vi "Tosca-2P Synchronization Simulator.vi"() -> ()   [LabVIEW 2020]
uses:
  <resource>/objmgr/daqmx.rc
  <vilib>/DAQmx/write.llb/DAQmx Write (Analog 2D DBL NChan NSamp).vi
  <vilib>/DAQmx/configure/timing.llb/DAQmx Timing (Sample Clock).vi
  <vilib>/DAQmx/create/channels.llb/DAQmx Create Channel (AO-Voltage-Basic).vi
  Signal Synthesis VIs/Waveform VIs/Pulse Train VIs/Pulse Polarity.ctl
  Signal Synthesis VIs/3rd Generation/Waveform VIs/Pulse Train VIs/Pulse Train.Properties.ctl
panel:
  in  "Nominal \"stim\" rate":dbl=1.0 format="%0.2f"
  in  "device":tag="PXI1Slot5"
  in  "Drift rate (us/s)":dbl format="%0.2f"
  in  "stop":bool
  in  "Buffer (s)":dbl=0.2 format="%0.2f"
  in  "Fs (Hz)":dbl=100000.0 format="%0.2f"
  in  "Pulse Train.Properties":T1={"Pulse width (us)"=10000.0, "Pulse rate (Hz)"=29.98, "Gap (ms)"=0.0, "Polarity"=enum."POS", "Asynch"=FALSE}
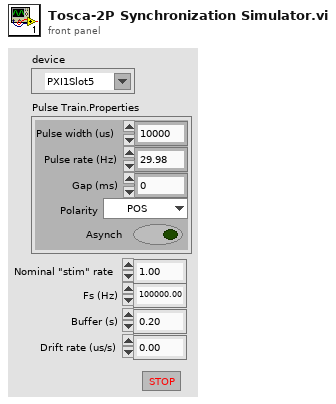
[diagram p1: front panel]
types:
  T1 = typedef "Pulse Train.Properties.ctl" = cluster{"Pulse width (us)":dbl, "Pulse rate (Hz)":dbl, "Gap (ms)":dbl, "Polarity":T2, "Asynch":bool}
  T2 = typedef "Pulse Polarity.ctl" = enum16{"POS", "NEG", "POS-NEG", "NEG-POS"}
  T3 = typedef "Pulse Train-Continuous State.ctl" = cluster{"Template":dbl[], "Nperiod":i32, "Index":i32, "Pulse Rate (Hz)":dbl, "Phase (cycles)":dbl, "Noff":i32}
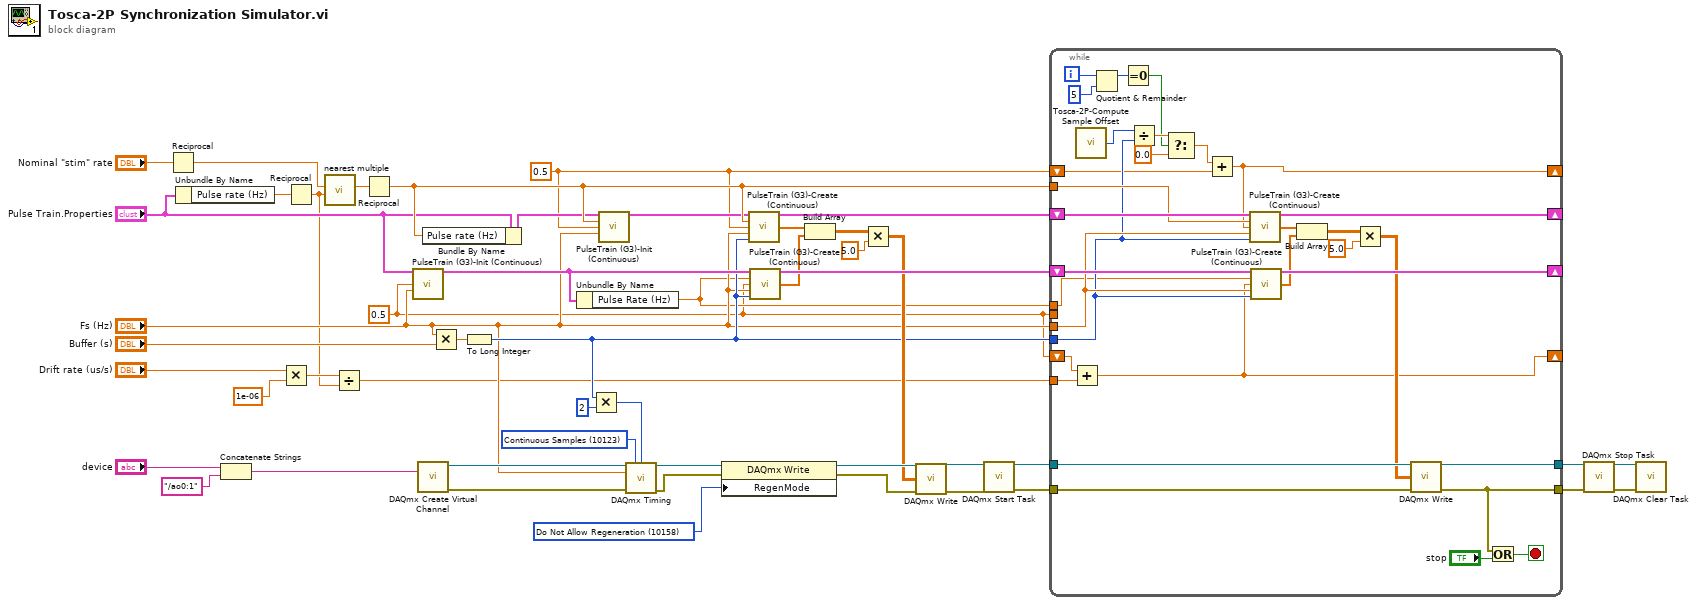
[diagram p0: block diagram]
diagram:
  w4 = 0.5 ("Start Phase (cycles)")
  w7 = 0.5 ("Start Phase (cycles)")
  w43 = 10158 items=["Allow Regeneration"=10097, "Do Not Allow Regeneration"=10158] ("RegenMode")
  w47 = 10123 items=["Finite Samples"=10178, "Continuous Samples"=10123, "Hardware Timed Single Point"=12522] ("sample mode")
  n1 = Reciprocal(x="Nominal \"stim\" rate") -> (1/x=w14:dbl)
  n2 = Unbundle By Name("Pulse Train.Properties") -> ("Pulse rate (Hz)"=w15:dbl)
  n3 = Concatenate Strings("device", "/ao0:1") -> (w23:string)
  n4 = Multiply(x="Drift rate (us/s)", y=1e-06) -> (x*y=w3:dbl)
  n5 = Reciprocal(x=w15) -> (1/x=w2:dbl)
  n6 = call "nearest multiple.vi"("y"=w2, "x"=w14) -> ("round(x/y)*y"=w13:dbl)  [unwired: 7 in, 2 out]
  n7 = Divide(x=w3, y=w2) -> (x/y=w1:dbl)
  n8 = Reciprocal(x=w13) -> (1/x=w12:dbl)
  n9 = call "PulseTrain (G3)-Init (Continuous).vi"("Pulse Train Params"="Pulse Train.Properties", "Start Phase (cycles)"=w4, "Fs (Hz)"="Fs (Hz)") -> ("Initial State"=w40:T3)  [unwired: 11 in, 1 out]
  n10 = call-poly <vilib>:"DAQmx Create Virtual Channel.vi"("physical channels"=w23) -> ("task out"=w49:refnum<k21>, "error out"=w48:errorcluster)  [unwired: 13 in]
  n11 = Bundle By Name(cluster="Pulse Train.Properties", "Pulse rate (Hz)"=w12) -> (w9:T1)
  n12 = Multiply(x="Fs (Hz)", y="Buffer (s)") -> (x*y=w46:dbl)
  n13 = To Long Integer(number=w46) -> (32bit integer=w17:i32)
  n14 = Unbundle By Name(w40) -> ("Pulse Rate (Hz)"=w6:dbl)
  n15 = Multiply(x=w17, y=2) -> (x*y=w30:i32)
  n16 = call "PulseTrain (G3)-Init (Continuous).vi"("Pulse Train Params"=w9, "Start Pulse Rate (Hz)"=w12, "Start Phase (cycles)"=w7, "Fs (Hz)"="Fs (Hz)") -> ("Initial State"=w11:T3)  [unwired: 10 in, 1 out]
  n17 = call-poly <vilib>:"DAQmx Timing.vi"("task/channels in"=w49, "sample mode"=w47, "samples per channel"=w30, "rate"="Fs (Hz)", "error in"=w48) -> ("task out"=w45:refnum<k21>, "error out"=w44:errorcluster)  [unwired: 9 in]
  n18 = property class="DAQmx Write"(reference=w45, error in=w44, "RegenMode"=w43) -> (reference out=w42:refnum<k21>, error out=w41:errorcluster)
  n19 = call "PulseTrain (G3)-Create (Continuous).vi"("State In"=w11, "Pulse Rate (Hz)"=w12, "Phase (cycles)"=w7, "Fs (Hz)"="Fs (Hz)", "Npts"=w17) -> ("State Out"=w21:T3, "Buffer"=w20:dbl[])  [unwired: 8 in, 1 out]
  n20 = call "PulseTrain (G3)-Create (Continuous).vi"("State In"=w40, "Pulse Rate (Hz)"=w6, "Phase (cycles)"=w4, "Fs (Hz)"="Fs (Hz)", "Npts"=w17) -> ("State Out"=w37:T3, "Buffer"=w19:dbl[])  [unwired: 8 in, 1 out]
  n21 = Build Array(w20, w19) -> (w18:dbl[][])
  n22 = Multiply(x=w18, y=5.0) -> (x*y=w28:dbl[][])
  n23 = call-poly <vilib>:"DAQmx Write.vi"("task/channels in"=w42, "data"=w28, "error in"=w41) -> ("task out"=w38:refnum<k21>, "error out"=w39:errorcluster)  [unwired: 10 in, 1 out]
  n24 = call <vilib>:"DAQmx Start Task.vi"("task/channels in"=w38, "error in"=w39) -> ("task out"=w35:refnum<k21>, "error out"=w36:errorcluster)  [unwired: 12 in]
  n25 = while {
    shift-right: [w79] -> _
    shift-left: w37 -> [w81]
    tunnel: w36 -> [w64]
    tunnel: w35 -> [w80]
    tunnel: "Fs (Hz)" -> [w69]
    tunnel: [w75] -> w33
    tunnel: [w78] -> w34
    tunnel: w17 -> [w63]
    shift-right: [w52] -> _
    shift-left: w4 -> [w72]
    shift-right: [w70] -> _
    shift-left: w21 -> [w71]
    tunnel: w12 -> [w65]
    shift-right: [w61] -> _
    shift-left: w7 -> [w62]
    tunnel: w4 -> [_]
    tunnel: w6 -> [w53]
    tunnel: w1 -> [w51]
    i -> [w60]
    stop <- w76 stop-if-true
    n26 = Add(x=w72, y=w51) -> (x+y=w52:dbl)
    n27 = call "Tosca-2P-Compute Sample Offset.vi"() -> ("Offset"=w54:i32)  [unwired: 13 in, 2 out]
    n28 = Quotient & Remainder(x=w60, y=5) -> (x-y*floor(x/y)=w58:i32)  [unwired: 1 out]
    n29 = Equal To 0?(x=w58) -> (x = 0?=w50:bool)
    n30 = Divide(x=w54, y=w63) -> (x/y=w57:dbl)
    n31 = Select(t=w57, s=w50, f=0.0) -> (s? t:f=w55:dbl)
    n32 = Add(x=w55, y=w62) -> (x+y=w61:dbl)
    n33 = call "PulseTrain (G3)-Create (Continuous).vi"("State In"=w71, "Pulse Rate (Hz)"=w65, "Phase (cycles)"=w61, "Fs (Hz)"=w69, "Npts"=w63) -> ("State Out"=w70:T3, "Buffer"=w68:dbl[])  [unwired: 8 in, 1 out]
    n34 = call "PulseTrain (G3)-Create (Continuous).vi"("State In"=w81, "Pulse Rate (Hz)"=w53, "Phase (cycles)"=w52, "Fs (Hz)"=w69, "Npts"=w63) -> ("State Out"=w79:T3, "Buffer"=w67:dbl[])  [unwired: 8 in, 1 out]
    n35 = Build Array(w68, w67) -> (w66:dbl[][])
    n36 = Multiply(x=w66, y=5.0) -> (x*y=w74:dbl[][])
    n37 = call-poly <vilib>:"DAQmx Write.vi"("task/channels in"=w80, "data"=w74, "error in"=w64) -> ("task out"=w78:refnum<k21>, "error out"=w75:errorcluster)  [unwired: 10 in, 1 out]
    n38 = Or(x=w75, y="stop") -> (x .or. y?=w76:bool)
  }
  n39 = call <vilib>:"DAQmx Stop Task.vi"("task/channels in"=w34, "error in"=w33) -> ("task out"=w32:refnum<k21>, "error out"=w31:errorcluster)  [unwired: 12 in]
  n40 = call <vilib>:"DAQmx Clear Task.vi"("task in"=w32, "error in"=w31) -> ()  [unwired: 13 in, 1 out]
